vi "Read Values.vi"(0 "Output in":refnum<class "Output.lvclass">) -> (7 "Output out":refnum<class "Output.lvclass">, 8 "Data Values":dbl[](array[numeric]), 10 "error out":errorcluster)   [LabVIEW 2018, in "Output.lvclass"]
doc: "Otput.lvclass:Write String.vi\n\nThis is the template for the Write String VI for the Output class.\n\nInstrument Communication Module Version 1.0\nOctober, 2020 Original Code Consulting Davita Bird\n www.originalcode.com"
uses:
  Output.lvclass
panel:
  in  "error out 2":errorcluster
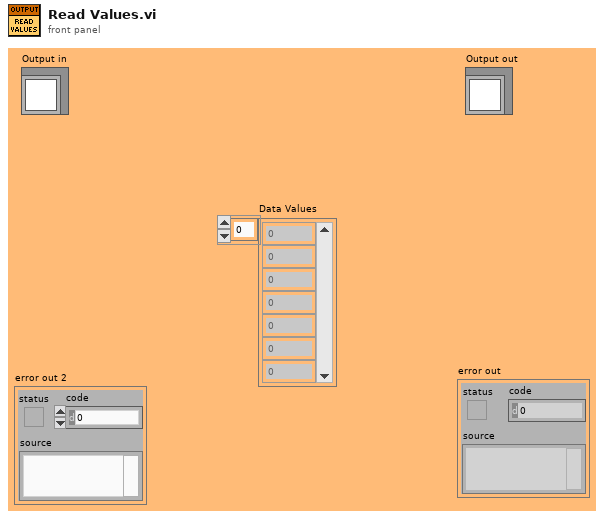
[diagram p1: front panel]
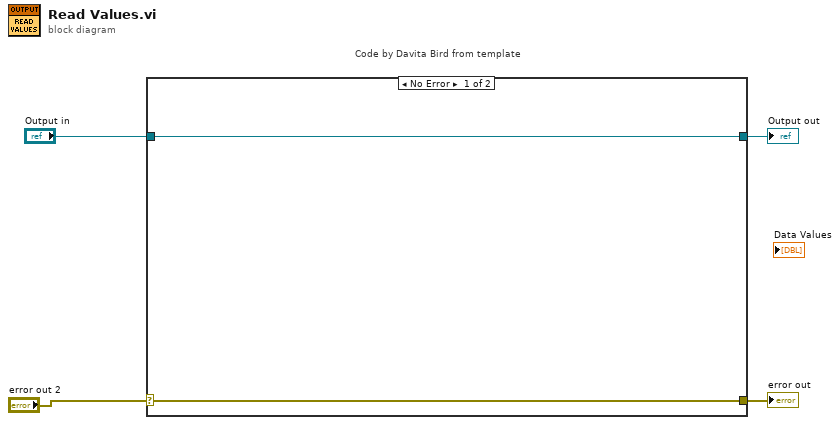
[diagram p0: block diagram]
diagram:
  n1 = case "Code by Davita Bird from template" shown="No Error" "error out 2" {
    selector: "error out 2" -> [w5 w8]
    tunnel: [w5 w8] -> w4
    tunnel: [w6 w7] -> w2
    tunnel: "Output in" -> [w6 w7]
    frame No Error {
    }
    frame Error {
    }
  }
  "error out" <- w4
  "Output out" <- w2
